vi "test_generic.vi"() -> ()   [LabVIEW 2010, in "GenericDetector.lvclass"]
uses:
  GenericDetector.lvclass
  common/classes/XMLElement/XMLElement/XMLElement.lvclass
  common/classes/GenericComponent/GenericComponent/GenericComponent.lvclass
panel:
  in  "generate OME XML button":bool
  in  "configure button":bool
  out "OME XML":string
  in  "create button":bool
  in  "stop":bool
  in  "enable button":bool
  in  "adjust button":bool
  # "Detector Test Program"
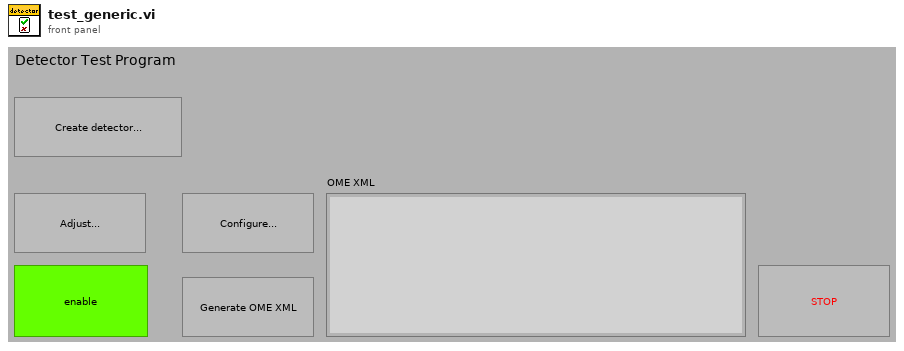
[diagram p1: front panel]
types:
  T1 = typedef "XComponentSpecification.xctl/data.ctl" = cluster{"class path":string, "configuration":string, "label":string, "settings name":string}
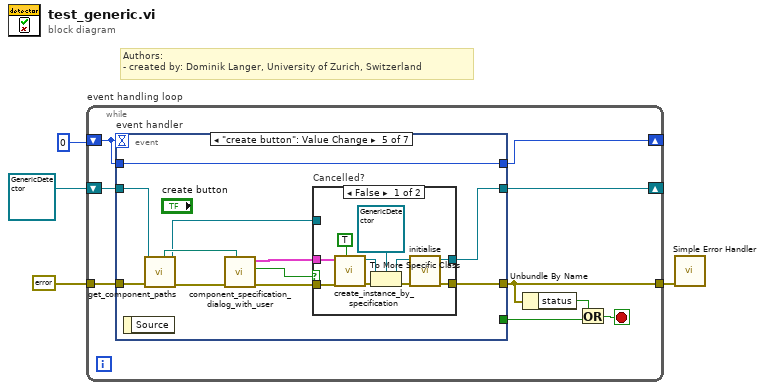
[diagram p0: block diagram]
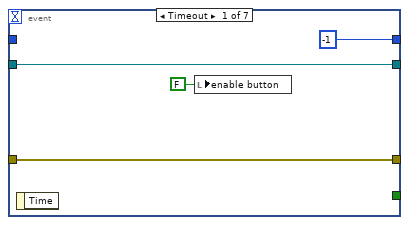
[diagram p2: hidden frame]
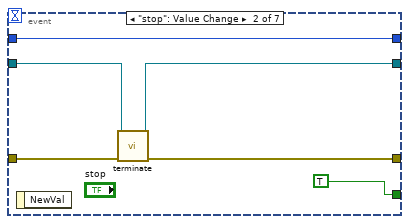
[diagram p3: hidden frame]
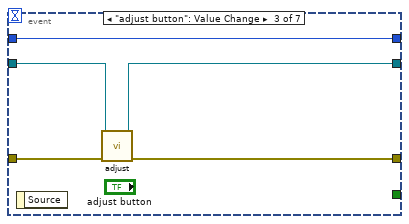
[diagram p4: hidden frame]
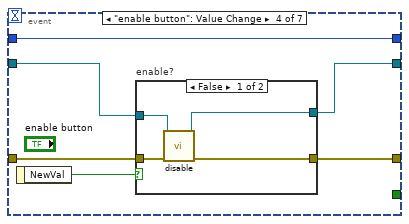
[diagram p5: hidden frame]
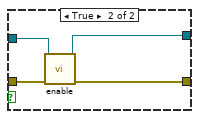
[diagram p6: hidden frame]
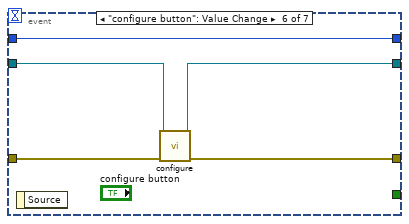
[diagram p8: hidden frame]
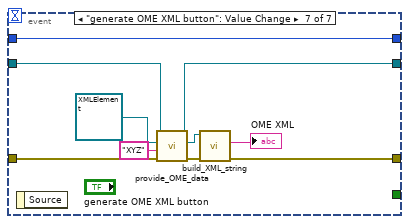
[diagram p9: hidden frame]
diagram:
  # "Authors: \n- created by: Dominik Langer, University of Zurich, Switzerland"
  n1 = while "event handling loop" {
    shift-right: [w11] -> _
    shift-left: 0 -> [w12]
    shift-right: [w10] -> _
    shift-left: refnum<class "GenericDetector.lvclass"> refnum ("GenericDetector.lvclass") -> [w9]
    tunnel: errorcluster {"status"=FALSE, "code"=0, "source"=""} ("error in (no error)") -> [w13]
    tunnel: [w8] -> w3
    stop <- w5 stop-if-true
    n2 = event "event handler" shown="[4] \"create button\": Value Change" {
      selector: _ -> [_ _ _ _ _ _ _]
      dyn-events: _ -> [_ _ _ _ _ _ _]
      timeout: w12 -> [_ _ _ _ _ _ _]
      tunnel: [w14 w20 w26 w31 w52 w66 w74] -> w8
      tunnel: w13 -> [w14 w21 w27 w33 w49 w67 w79]
      tunnel: [_ TRUE _ _ _ _ _] -> w7
      tunnel: [-1 w22 w28 w34 w53 w70 w80] -> w11
      tunnel: w12 -> [_ w22 w28 w34 w53 w70 w80]
      tunnel: [w15 w18 w24 w29 w45 w68 w77] -> w10
      tunnel: w9 -> [w15 w19 w25 w30 w47 w69 w78]
      event Timeout {
        n3 = event-data() -> ()  [unwired: 2 out]
        n4 = local write "enable button"(FALSE ("enable button")) -> ()
      }
      event "stop": Value Change {
        n5 = event-data() -> ()  [unwired: 2 out]
        n6 = call-dynamic "terminate.vi"("error in (no error)"=w21, "GenericPlugin in"=w19) -> ("error out"=w20:errorcluster, "GenericPlugin out"=w18:refnum<class "GenericDetector.lvclass">)  [unwired: 8 out]
      }
      event "adjust button": Value Change {
        n7 = event-data() -> ()  [unwired: 2 out]
        n8 = call-dynamic "adjust.vi"("error in (no error)"=w27, "GenericEmissionSensor in"=w25) -> ("error out"=w26:errorcluster, "GenericEmissionSensor out"=w24:refnum<class "GenericDetector.lvclass">)  [unwired: 8 out]
      }
      event "enable button": Value Change {
        n9 = event-data() -> ("NewVal"=w32:bool)  [unwired: 1 out]
        n10 = case "enable?" shown="False" w32 {
          tunnel: w33 -> [w38 w42]
          tunnel: [w37 w41] -> w31
          tunnel: [w36 w40] -> w29
          tunnel: w30 -> [w35 w39]
          frame False {
            n11 = call-dynamic "disable.vi"("error in (no error)"=w38, "GenericEmissionSensor in"=w35) -> ("error out"=w37:errorcluster, "GenericEmissionSensor out"=w36:refnum<class "GenericDetector.lvclass">)  [unwired: 8 out]
          }
          frame True {
            n12 = call-dynamic "enable.vi"("error in (no error)"=w42, "GenericEmissionSensor in"=w39) -> ("error out"=w41:errorcluster, "GenericEmissionSensor out"=w40:refnum<class "GenericDetector.lvclass">)  [unwired: 8 out]
          }
        }
      }
      event "create button": Value Change {
        n13 = event-data() -> ()  [unwired: 2 out]
        n14 = call-dynamic "get_component_paths.vi"("error in (no error)"=w49, "GenericComponent in"=w47) -> ("error out"=w50:errorcluster, "GenericComponent out"=w43:refnum<class "GenericDetector.lvclass">, "component type directory"=w51:path)  [unwired: 4 in, 3 out]
        n15 = call "component_specification_dialog_with_user.vi"("start path"=w51, "error in (no error)"=w50) -> ("error out"=w48:errorcluster, "cancelled?"=w44:bool, "component specification out"=w46:T1)  [unwired: 7 in]
        n16 = case "Cancelled?" shown="False" w44 {
          tunnel: [w62 w65] -> w52
          tunnel: w48 -> [w56 w65]
          tunnel: w46 -> [w55 _]
          tunnel: [w54 w64] -> w45
          tunnel: w43 -> [_ w64]
          frame False {
            n17 = call "create_instance_by_specification.vi"("call constructor?"=TRUE, "error in (no error)"=w56, "component specification"=w55) -> ("error out"=w59:errorcluster, "GenericPlugin out"=w58:refnum<class "GenericComponent.lvclass">)  [unwired: 6 in, 1 out]
            n18 = To More Specific Class(target class=refnum<class "GenericDetector.lvclass"> refnum ("GenericEmissionSensor.lvclass"), reference=w58, error in=w59) -> (specific class reference=w60:refnum<class "GenericDetector.lvclass">, error out=w61:errorcluster)
            n19 = call-dynamic "initialise.vi"("error in (no error)"=w61, "GenericPlugin in"=w60) -> ("error out"=w62:errorcluster, "GenericPlugin out"=w54:refnum<class "GenericDetector.lvclass">)  [unwired: 8 out]
          }
          frame True {
          }
        }
      }
      event "configure button": Value Change {
        n20 = event-data() -> ()  [unwired: 2 out]
        n21 = call-dynamic "configure.vi"("error in (no error)"=w67, "GenericPlugin in"=w69) -> ("error out"=w66:errorcluster, "GenericPlugin out"=w68:refnum<class "GenericDetector.lvclass">)  [unwired: 8 in]
      }
      event "generate OME XML button": Value Change {
        n22 = event-data() -> ()  [unwired: 2 out]
        n23 = call-dynamic "provide_OME_data.vi"("error in (no error)"=w79, "structuredAttribute string in"="XYZ" ("image ID"), "OME element in"=refnum<class "XMLElement.lvclass"> refnum ("XMLElement.lvclass"), "GenericPlugin in"=w78) -> ("error out"=w76:errorcluster, "OME element out"=w75:refnum<class "XMLElement.lvclass">, "GenericPlugin out"=w77:refnum<class "GenericDetector.lvclass">)  [unwired: 4 in, 1 out]
        n24 = call "build_XML_string.vi"("error in (no error)"=w76, "Element in"=w75) -> ("error out"=w74:errorcluster, "string"=→"OME XML":string)  [unwired: 7 in, 1 out]
      }
    }
    n25 = Unbundle By Name(w8) -> ("status"=w6:bool)
    n26 = Or(x=w6, y=w7) -> (x .or. y?=w5:bool)
  }
  n27 = call <vilib>:"Simple Error Handler.vi"("error in (no error)"=w3) -> ()  [unwired: 1 in, 8 out]
